vi "initiate.vi"(8 "error in (no error)":errorcluster, 11 "reference in":refnum<class "Project Panels.lvclass">) -> (0 "error out":errorcluster, 3 "reference out":refnum<class "Project Panels.lvclass">)   [LabVIEW 2015, in "Project Panels.lvclass"]
uses:
  Project Panels.lvclass
  SYS/File Controller_llb/File Controller.lvclass
  SYS/Subject Controller_llb/Subject Controller.lvclass
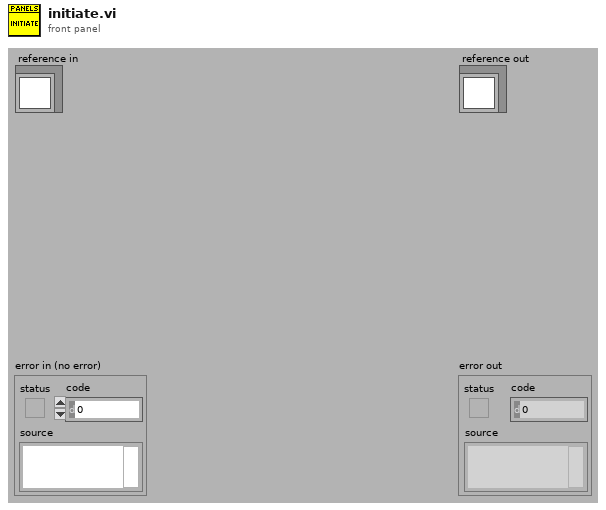
[diagram p1: front panel]
types:
  T1 = typedef "Project Panels.lvclass/ObjectAttributesRef.ctl" = refnum<data-value>
  T2 = typedef "Project Panels.lvclass/ObjectAttributes.ctl" = cluster{"MyAttribute":dbl, "file_controller_ref":refnum<class "File Controller.lvclass">, "subject_controller_ref":refnum<class "Subject Controller.lvclass">}
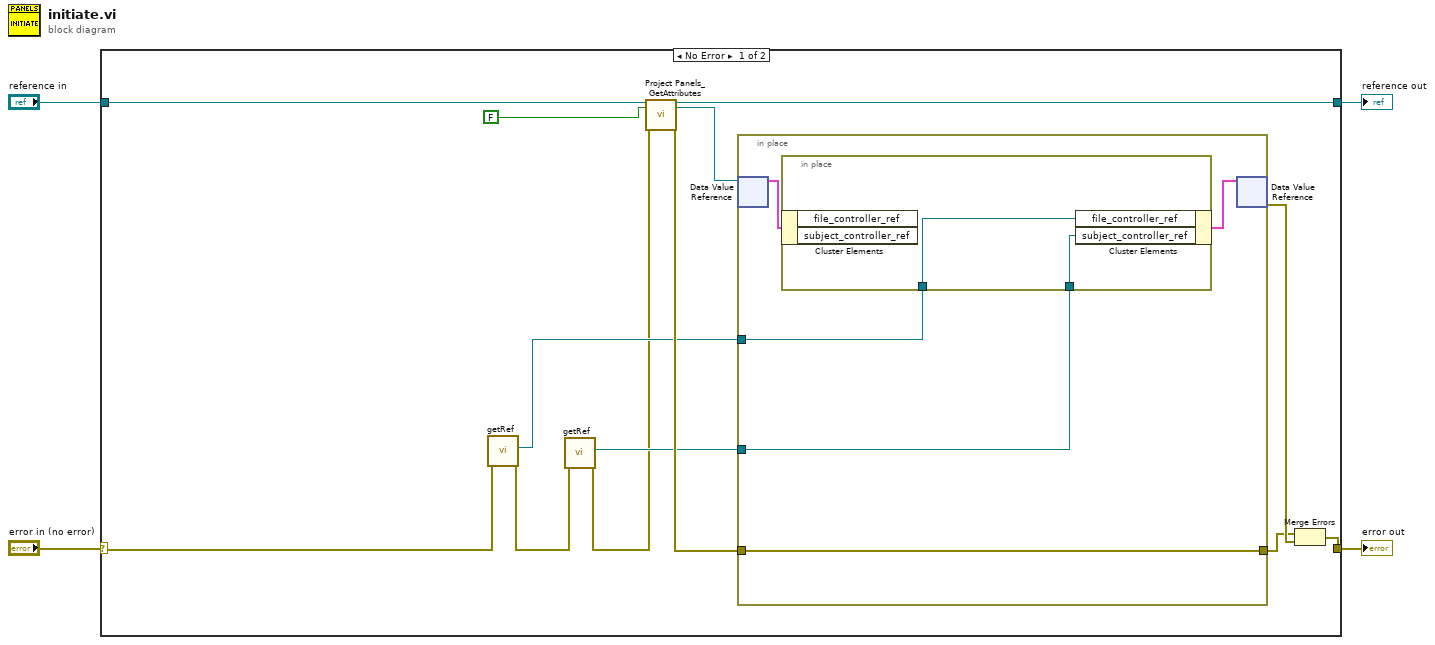
[diagram p0: block diagram]
diagram:
  n1 = case shown="No Error" "error in (no error)" {
    selector: "error in (no error)" -> [w9 w26]
    tunnel: [w17 w26] -> w3
    tunnel: [w11 w25] -> w1
    tunnel: "reference in" -> [w14 w25]
    frame No Error {
      n2 = call "getRef.vi"("error in (no error)"=w9) -> ("error out"=w6:errorcluster, "File Controller.lvclass"=w8:refnum<class "File Controller.lvclass">)  [unwired: 9 in]
      n3 = call "getRef.vi"("error in (no error)"=w6) -> ("error out"=w5:errorcluster, "subject_controller_ref"=w7:refnum<class "Subject Controller.lvclass">)  [unwired: 9 in]
      n4 = call "Project Panels_GetAttributes.vi"("reference in"=w14, "return data? (T)"=FALSE, "error in (no error)"=w5) -> ("reference out"=w11:refnum<class "Project Panels.lvclass">, "attributes ref"=w10:T1, "error out"=w12:errorcluster)  [unwired: 13 in, 1 out]
      n5 = in-place {
        in-place-border: w12 -> [w20]
        in-place-border: [w20] -> w15
        in-place-border: w8 -> [w19]
        in-place-border: w7 -> [w18]
        n6 = in-place-dvr #1(w10) -> (w21:T2)  [unwired: 1 out]
        n7 = in-place {
          in-place-border: w19 -> [w24]
          in-place-border: w18 -> [w23]
          n8 = in-place-cluster #2(w21) -> ()  [unwired: 2 out]
          n9 = in-place-cluster #2("file_controller_ref"=w24, "subject_controller_ref"=w23) -> (w22:T2)
        }
        n10 = in-place-dvr #1(w22) -> (w16:errorcluster)  [unwired: 1 out]
      }
      n11 = Merge Errors(w15, w16) -> (w17:errorcluster)
    }
    frame Error {
    }
  }
  "error out" <- w3
  "reference out" <- w1
